vi "Play Sound.vi"() -> ()   [LabVIEW 2023]
panel:
  in  "Device ID":u32
  out "Sound Is Playing?":bool
  in  "Stop":bool
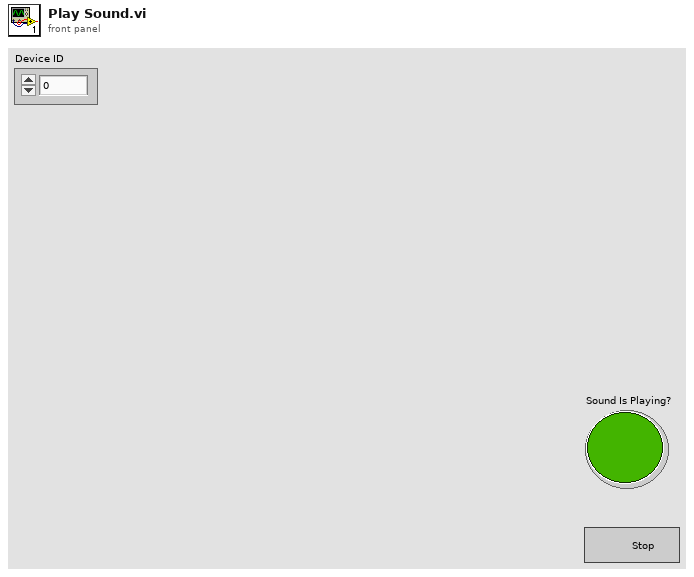
[diagram p1: front panel]
types:
  T1 = typedef "Sound Output Task ID.ctl" = u32
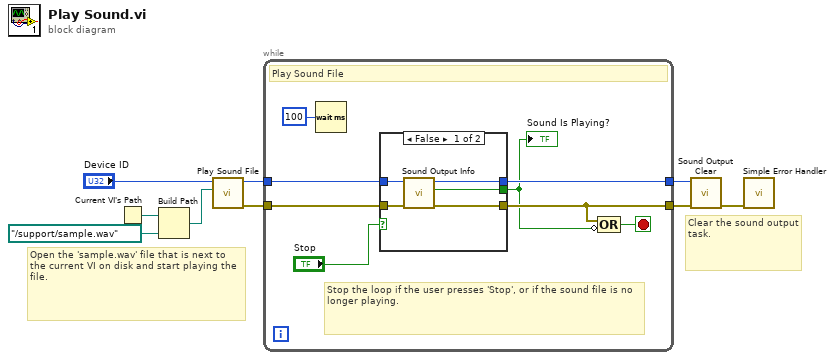
[diagram p0: block diagram]
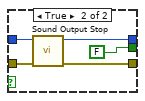
[diagram p2: hidden frame]
diagram:
  # "Clear the sound output task."
  # "Open the 'sample.wav' file that is next to the current VI on disk and start playing the file."
  n1 = Current VI's Path() -> (path=w1:path)
  n2 = Build Path(base path=w1, name or relative path=path "../support/sample.wav" ("Sound File Path")) -> (appended path=w2:path)
  n3 = call <vilib>:"Play Sound File.vi"("path"=w2, "device ID"="Device ID") -> ("error out"=w8:errorcluster, "task ID"=w9:T1)  [unwired: 8 in]
  n4 = while {
    tunnel: w9 -> [w11]
    tunnel: [w16] -> w6
    tunnel: w8 -> [w12]
    tunnel: [w15] -> w7
    stop <- w17 stop-if-true
    # "Stop the loop if the user presses 'Stop', or if the sound file is no longer playing."
    # "Play Sound File"
    n5 = Wait (ms)(milliseconds to wait=u32 100) -> ()  [unwired: 1 out]
    n6 = case shown="False" "Stop" {
      tunnel: w12 -> [w22 w26]
      tunnel: [w21 w24] -> w16
      tunnel: w11 -> [w20 w27]
      tunnel: [w19 w25] -> w15
      tunnel: [w18 FALSE] -> w14
      frame False {
        n7 = call <vilib>:"Sound Output Info.vi"("error in (no error)"=w22, "task ID"=w20) -> ("error out"=w19:errorcluster, "is playing?"=w18:bool, "task ID out"=w21:T1)  [unwired: 6 in, 1 out]
      }
      frame True {
        n8 = call <vilib>:"Sound Output Stop.vi"("error in (no error)"=w26, "task ID"=w27) -> ("error out"=w25:errorcluster, "task ID out"=w24:T1)  [unwired: 8 in]
      }
    }
    "Sound Is Playing?" <- w14
    n9 = Compound Arithmetic op=OR(w15, invert w14) -> (w17:bool)
  }
  n10 = call <vilib>:"Sound Output Clear.vi"("error in (no error)"=w7, "task ID"=w6) -> ("error out"=w4:errorcluster)  [unwired: 9 in]
  n11 = call <vilib>:"Simple Error Handler.vi"("error in (no error)"=w4) -> ()  [unwired: 4 in, 5 out]
